vi "Error Process.vi"(8 "error in (no error)":errorcluster, 11 "View Model":T1) -> (0 "error out":errorcluster, 3 "View Model":T1)   [LabVIEW 2017]
doc: "Centralized error handler of ATM controller"
uses:
  View Model/Controls/View Model.ctl
  Controls/Error Model.ctl
  Controls/Error Data.ctl
  Controls/Error Type.ctl
  View Model/Controls/Shared Model.ctl
  Configuration/Controls/Config Model.ctl
  Configuration/Controls/Config CMD.ctl
  Configuration/Controls/Config Data.ctl
  ATM Controller/Controls/Controller Model.ctl
  ATM Controller/Controls/Controller Overhead.ctl
  ATM Controller/Controls/Controller States.ctl
  ATM Controller/Controls/Controller Message Data.ctl
  ATM Controller/Controls/Controller Message Name.ctl
  Views/User Console View/Controls/User Console - Keypad.ctl
  Views/User Console View/Controls/User Console - Transactions.ctl
  ATM Controller/Controls/Controller CMD.ctl
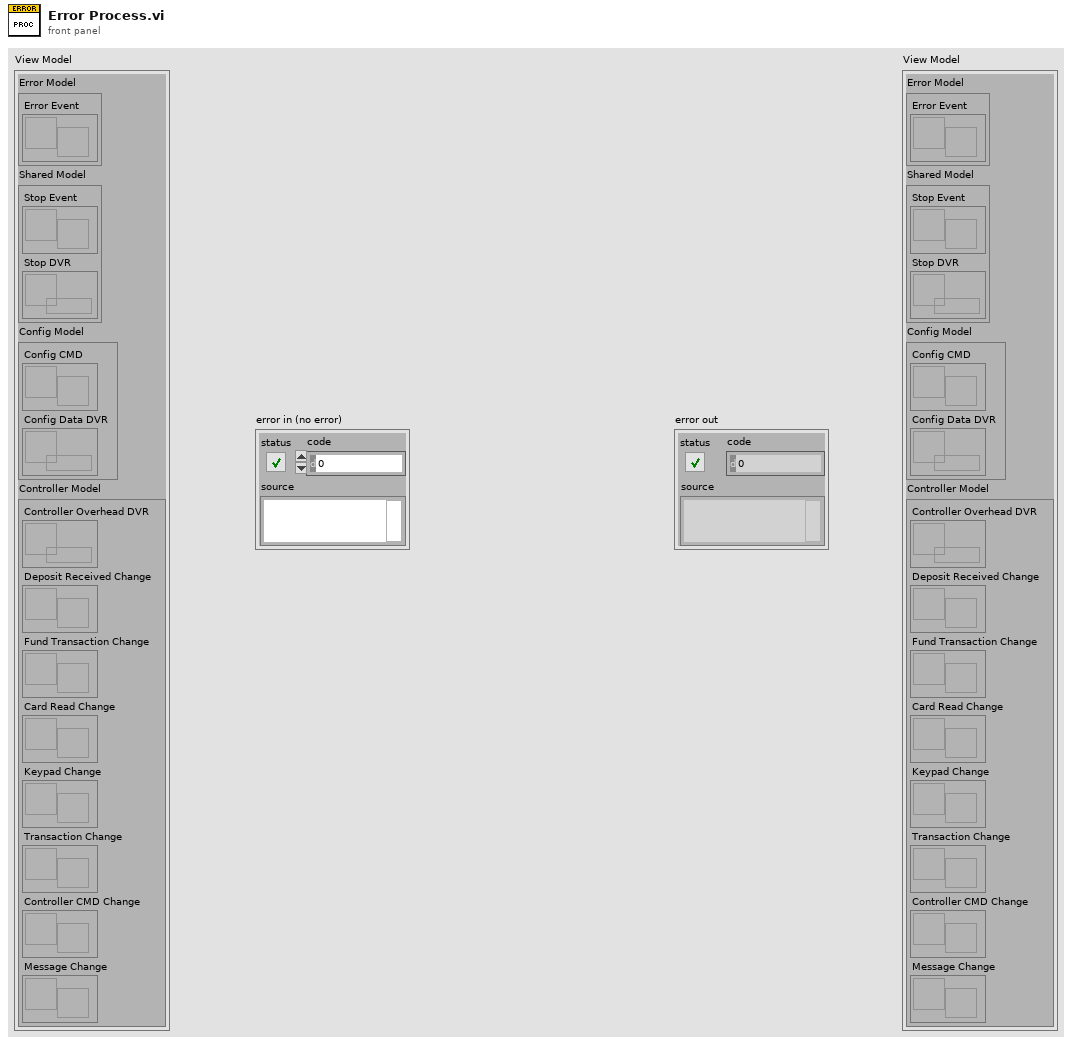
[diagram p1: front panel]
types:
  T1 = typedef "View Model.ctl" = cluster{"Error Model":T2, "Shared Model":T3, "Config Model":T4, "Controller Model":T5}
  T2 = typedef "Error Model.ctl" = cluster{"Error Event":refnum<user-event>}
  T3 = typedef "Shared Model.ctl" = cluster{"Stop Event":refnum<user-event>, "Stop DVR":refnum<data-value>}
  T4 = typedef "Config Model.ctl" = cluster{"Config CMD":refnum<user-event>, "Config Data DVR":refnum<data-value>}
  T5 = typedef "Controller Model.ctl" = cluster{"Controller Overhead DVR":refnum<data-value>, "Deposit Received Change":refnum<user-event>, "Fund Transaction Change":refnum<user-event>, "Card Read Change":refnum<user-event>, "Keypad Change":refnum<user-event>, "Transaction Change":refnum<user-event>, "Controller CMD Change":refnum<user-event>, "Message Change":refnum<user-event>}
  T6 = typedef "Error Data.ctl" = cluster{"Error Type":T7, "Variant":variant}
  T7 = typedef "Error Type.ctl" = enum16{"Console Error", "Sensor Interface IO Error", "Process Step Error"}
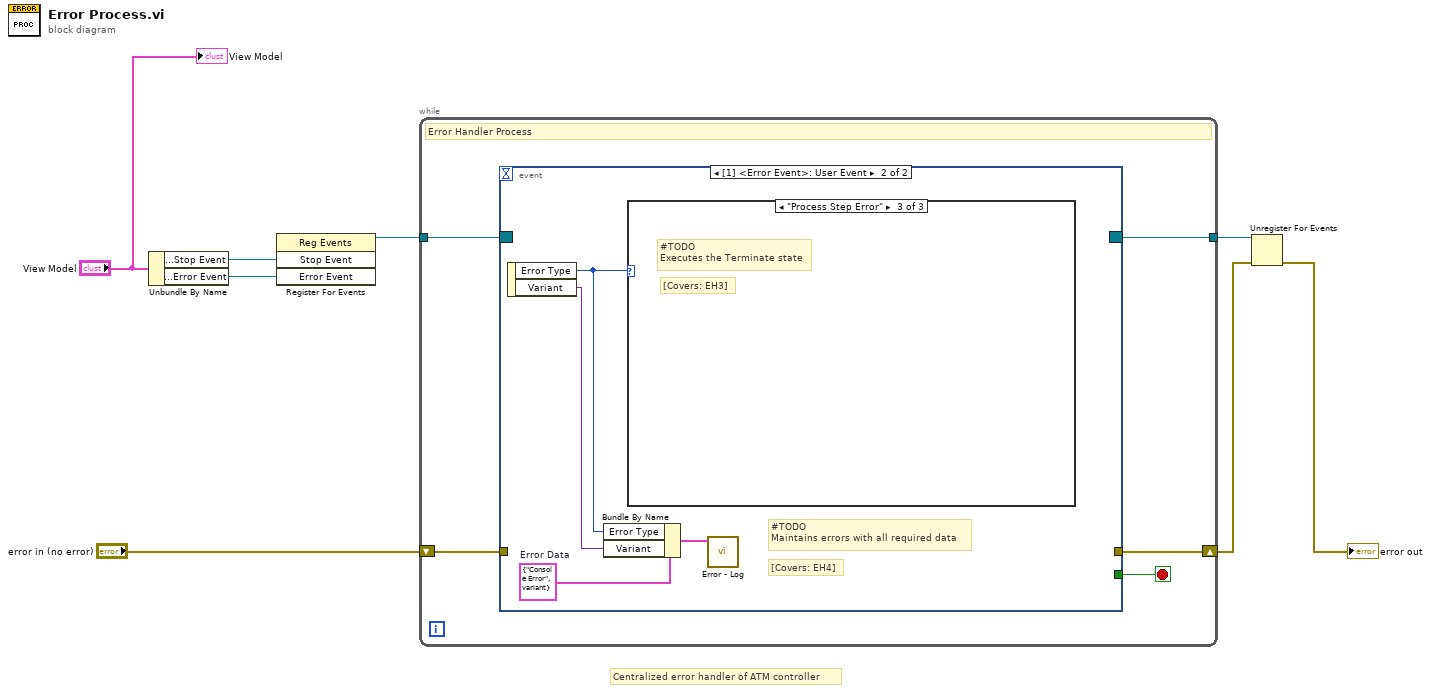
[diagram p0: block diagram]
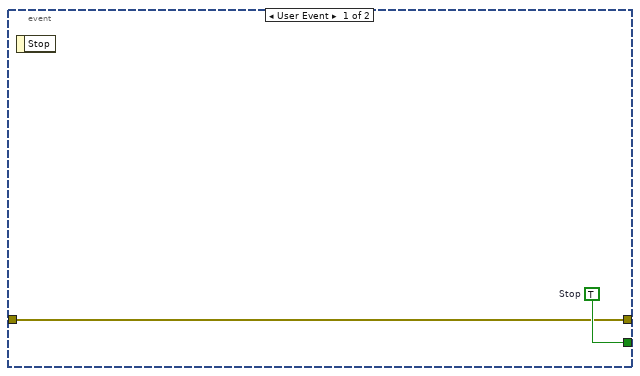
[diagram p2: hidden frame]
diagram:
  # "Centralized error handler of ATM controller"
  n1 = Unbundle By Name("View Model") -> ("Shared Model.Stop Event"=w8:refnum<user-event>, "Error Model.Error Event"=w1:refnum<user-event>)
  n2 = register-events(w8, w1) -> (reference out=w7:refnum<event-registration>)  [unwired: 2 in, 1 out]
  n3 = while {
    tunnel: w7 -> [w13]
    shift-right: [w10] -> w3
    shift-left: "error in (no error)" -> [w11]
    tunnel: [w9] -> w4
    stop <- w12 stop-if-true
    # "Error Handler Process"
    n4 = event shown="[1] <Error Event>: User Event" {
      selector: w13 -> [_ _]
      dyn-events: [_ _] -> w9
      timeout: _ -> [_ _]
      tunnel: [w15 _] -> w12
      tunnel: w11 -> [w14 _]
      tunnel: [w14 _] -> w10
      event User Event {
        w15 = TRUE  # Stop
        n5 = event-data() -> ()  [unwired: 1 in, 1 out]
      }
      event User Event {
        w19 = T6 {"Error Type"=enum."Console Error", "Variant"=variant}  # Error Data
        # "[Covers: EH4]"
        # "#TODO\nMaintains errors with all required data"
        n6 = event-data() -> ("Error Type"=w17:T7, "Variant"=w18:variant)  [unwired: 1 in]
        n7 = Bundle By Name(cluster=w19, "Error Type"=w17, "Variant"=w18) -> (w16:T6)
        n8 = case shown="\"Process Step Error\"" w17 {
          frame "Console Error", Default {
            # "[Covers: EH1B2]"
            # "[Covers: EH1B1]"
            # "[Covers: EH1B]"
            # "[Covers: EH1A]"
            # "Check If an error occurs in User Console user should choose by dialog,\nto clear error and continue last operation OR continue with error and \nhandle it as a Process Step Error"
            # "Check If an error occurs in Display Console notify user by dialog, clear error\nand continue las operation/step."
            # "[Covers: EH1]"
            # "#TODO\nNotify user about error and continue work without interuption"
          }
          frame "Sensor Interface IO Error" {
            # "[Covers: EH2]"
            # "#TODO\nExecutes the Terminate state"
          }
          frame "Process Step Error" {
            # "[Covers: EH3]"
            # "#TODO\nExecutes the Terminate state"
          }
        }
        n9 = call "Error - Log.vi"("Error Data"=w16) -> ()  [unwired: 10 in, 1 out]
      }
    }
  }
  n10 = Unregister For Events(event registration refnum=w4, error in=w3) -> (error out=→"error out":errorcluster)
  "View Model" <- "View Model"
